vi "Boiler-M.vi"() -> ()   [LabVIEW 2020]
uses:
  Controls/Boiler States Enum-M.ctl
panel:
  in  "stop":bool
  out "Boiler Status Indicators":T1 {"Time Count" format="%.2f"}
  in  "Boiler Simulation Controls":T2 {"Flame Sesnor Value (%)" scale=0.0..100.0}
  in  "Boiler Controls":T3 {"Fuel Control Valve Position (% Open)" scale=0.0..100.0 scale format="%_3g"}
  # "Seconds"
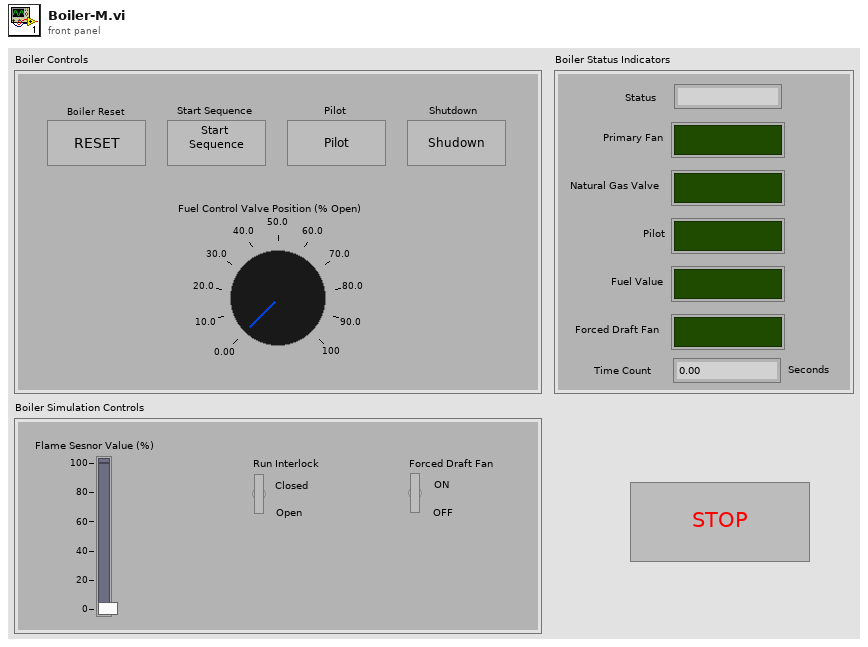
[diagram p1: front panel]
types:
  T1 = cluster{"Primary Fan":bool, "Natural Gas Valve":bool, "Pilot":bool, "Fuel Value":bool, "Forced Draft Fan":bool, "Time Count    ":dbl, "Status":string}
  T2 = cluster{"Flame Sesnor Value (%)":dbl, "Run Interlock":bool, "Forced Draft Fan":bool}
  T3 = cluster{"Shutdown":bool, "Pilot":bool, "Start Sequence":bool, "Fuel Control Valve Position (% Open)":dbl, "Boiler Reset":bool}
  T4 = typedef "Boiler States Enum-M.ctl" = enum16{"Idle", "Initialize", "Reset Lockout", "Pre-Purge", "Pre-Purge Complete", "Ignition", "Pilot", "Shutdown Purge Complete", "Shutdown Purge Start", "Run", "Pilot Proved", "Forced Draft Fan On"}
  T5 = cluster{"Time has Elapsed":bool, "Elapsed Time (s)":dbl}
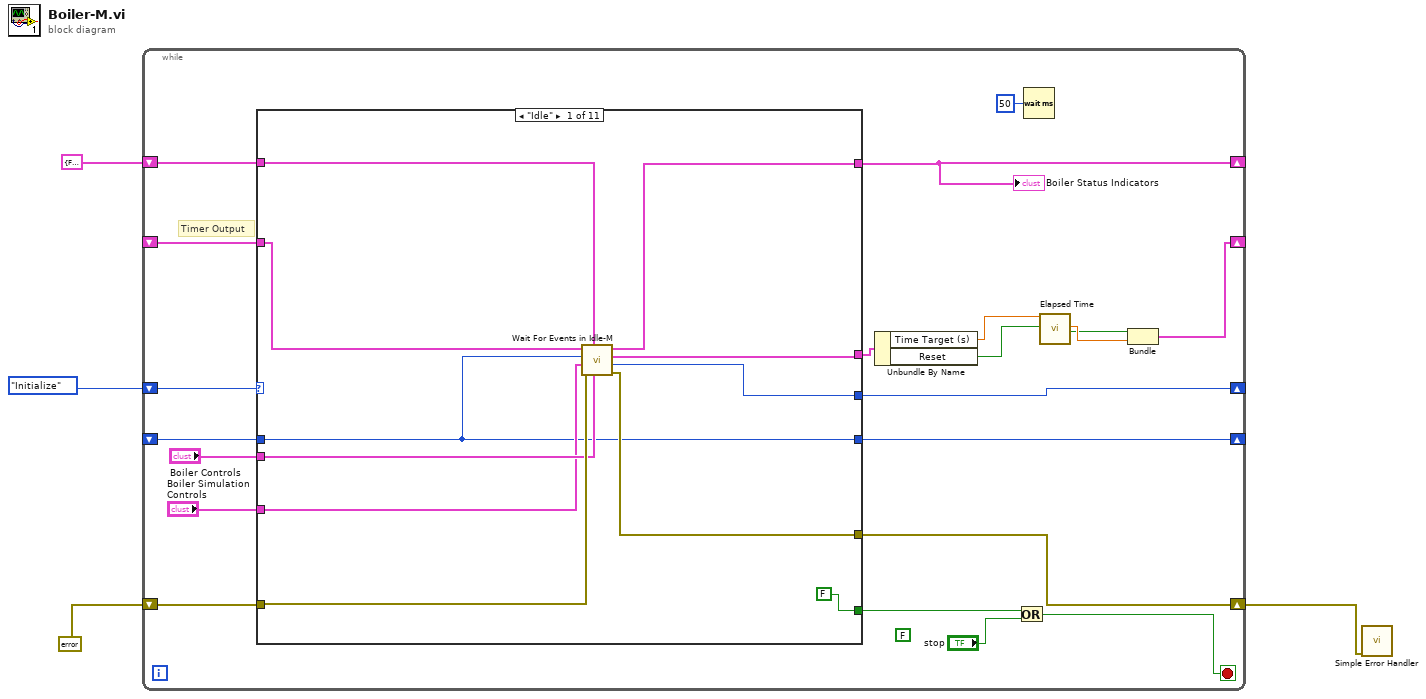
[diagram p0: block diagram]
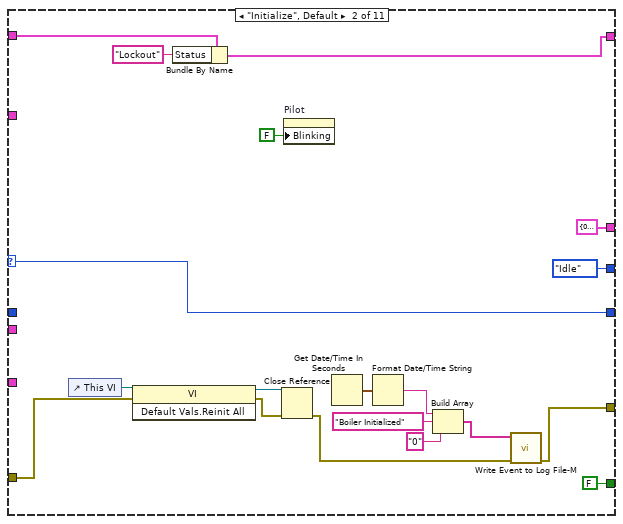
[diagram p2: hidden frame]
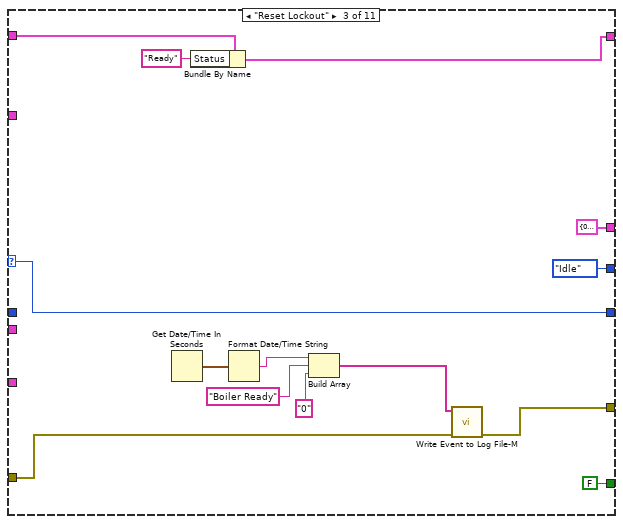
[diagram p3: hidden frame]
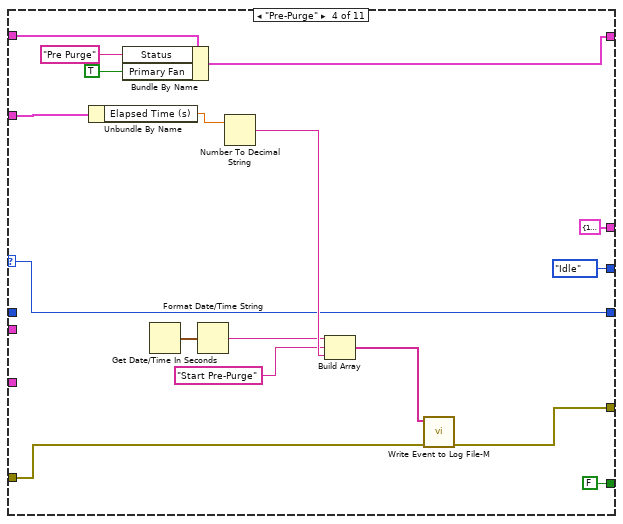
[diagram p4: hidden frame]
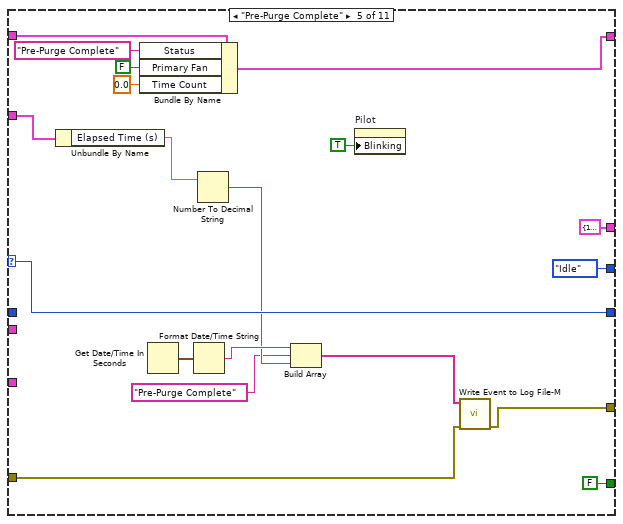
[diagram p5: hidden frame]
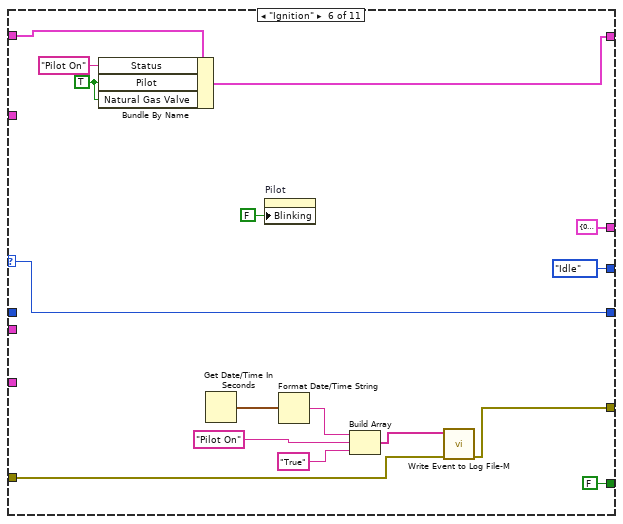
[diagram p6: hidden frame]
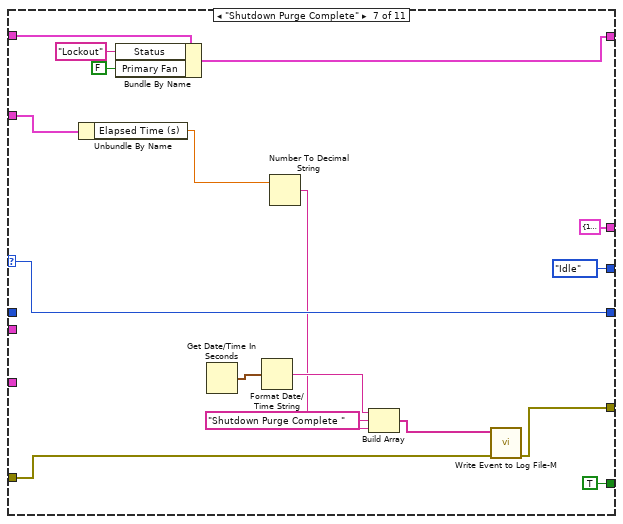
[diagram p7: hidden frame]
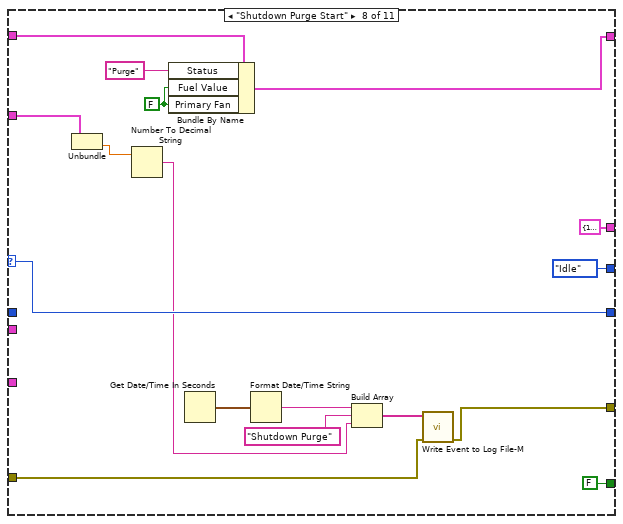
[diagram p8: hidden frame]
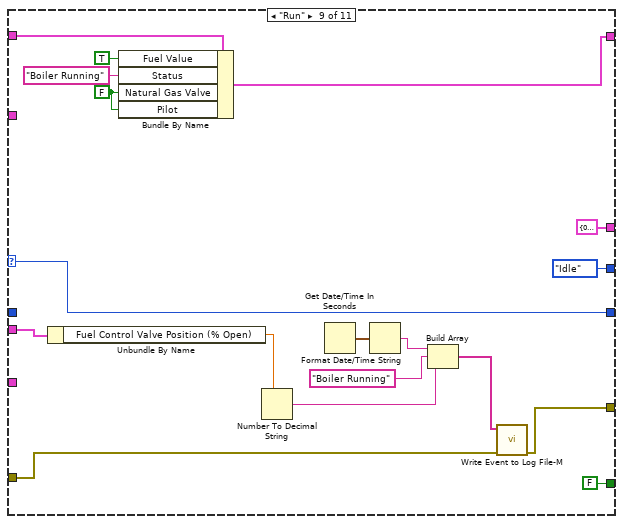
[diagram p9: hidden frame]
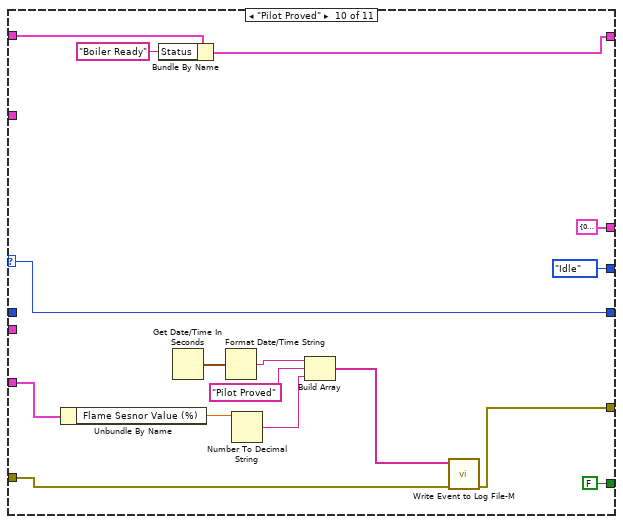
[diagram p10: hidden frame]
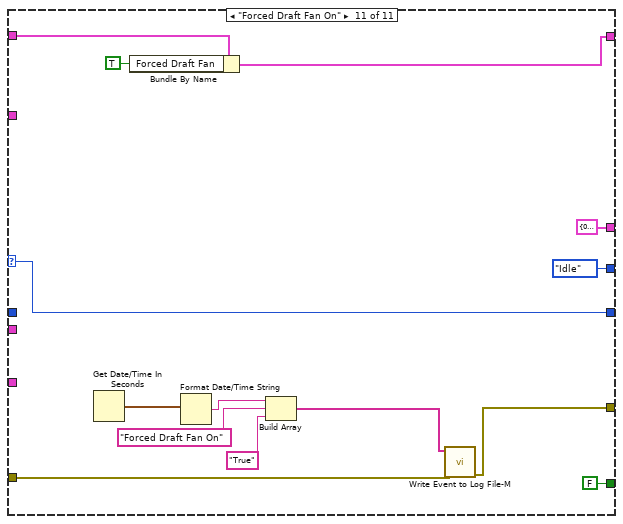
[diagram p11: hidden frame]
diagram:
  n1 = while {
    shift-right: [w24] -> _
    shift-left: T1 {"Primary Fan"=FALSE, "Natural Gas Valve"=FALSE, "Pilot"=FALSE, "Fuel Value"=FALSE, "Forced Draft Fan"=FALSE, "Time Count    "=0.0, "Status"=""} ("Boiler Status Indicators") -> [w25]
    shift-right: [w19] -> _
    shift-left: _ -> [w10]
    shift-right: [w13] -> _
    shift-left: Boiler_States_Enum-M."Initialize" ("Enum") -> [w14]
    shift-right: [w8] -> _
    shift-left: _ -> [w7]
    shift-right: [w9] -> w1
    shift-left: errorcluster {"status"=FALSE, "code"=0, "source"=""} ("error in (no error)") -> [w15]
    stop <- w18 stop-if-true
    (unwired) FALSE
    # "Timer Output"
    n2 = case shown="\"Idle\"" w14 {
      selector: w14 -> [_ w55 w64 w74 w104 w114 w138 w149 w160 w186 w199]
      tunnel: w25 -> [w36 w53 w69 w86 w102 w121 w125 w155 w163 w189 w203]
      tunnel: [w35 w52 w68 w83 w101 w107 w124 w154 w162 w188 w202] -> w24
      tunnel: [w34 cluster{"Time Target (s)":dbl, "Reset":bool} {"Time Target (s)"=0.0, "Reset"=TRUE} ("Cluster out") cluster{"Time Target (s)":dbl, "Reset":bool} {"Time Target (s)"=0.0, "Reset"=TRUE} ("Cluster out") cluster{"Time Target (s)":dbl, "Reset":bool} {"Time Target (s)"=10.0, "Reset"=TRUE} ("Cluster out") cluster{"Time Target (s)":dbl, "Reset":bool} {"Time Target (s)"=10.0, "Reset"=TRUE} ("Cluster out") cluster{"Time Target (s)":dbl, "Reset":bool} {"Time Target (s)"=0.0, "Reset"=TRUE} ("Cluster out") cluster{"Time Target (s)":dbl, "Reset":bool} {"Time Target (s)"=10.0, "Reset"=TRUE} ("Cluster out") cluster{"Time Target (s)":dbl, "Reset":bool} {"Time Target (s)"=10.0, "Reset"=TRUE} ("Cluster out") cluster{"Time Target (s)":dbl, "Reset":bool} {"Time Target (s)"=0.0, "Reset"=TRUE} ("Cluster out") cluster{"Time Target (s)":dbl, "Reset":bool} {"Time Target (s)"=0.0, "Reset"=TRUE} ("Cluster out") cluster{"Time Target (s)":dbl, "Reset":bool} {"Time Target (s)"=0.0, "Reset"=TRUE} ("Cluster out")] -> w22
      tunnel: [FALSE FALSE FALSE FALSE FALSE FALSE TRUE FALSE FALSE FALSE FALSE] -> w16
      tunnel: [w32 w46 w57 w80 w91 w115 w134 w146 w169 w178 w195] -> w9
      tunnel: w15 -> [w31 w49 w63 w79 w90 w116 w133 w140 w167 w179 w196]
      tunnel: [w30 Boiler_States_Enum-M."Idle" ("Next State") Boiler_States_Enum-M."Idle" ("Next State") Boiler_States_Enum-M."Idle" ("Next State") Boiler_States_Enum-M."Idle" ("Next State") Boiler_States_Enum-M."Idle" ("Next State") Boiler_States_Enum-M."Idle" ("Next State") Boiler_States_Enum-M."Idle" ("Next State") Boiler_States_Enum-M."Idle" ("Next State") Boiler_States_Enum-M."Idle" ("Next State") Boiler_States_Enum-M."Idle" ("Next State")] -> w13
      tunnel: "Boiler Controls" -> [w29 _ _ _ _ _ _ _ w172 _ _]
      tunnel: "Boiler Simulation Controls" -> [w28 _ _ _ _ _ _ _ _ w183 _]
      tunnel: w10 -> [w26 _ _ w82 w98 _ w137 w148 _ _ _]
      tunnel: [w27 w55 w64 w74 w104 w114 w138 w149 w160 w186 w199] -> w8
      tunnel: w7 -> [w27 _ _ _ _ _ _ _ _ _ _]
      frame "Idle" {
        n3 = call "Wait For Events in Idle-M.vi"("Boiler Controls"=w29, "Boiler Status Indicators In"=w36, "error in (no error)"=w31, "Boiler Simulation Controls"=w28, "Last State Before Idle"=w27, "Timer Ouput"=w26) -> ("error out"=w32:errorcluster, "Next State"=w30:T4, "Cluster out"=w34:cluster{"Time Target (s)":dbl, "Reset":bool}, "Boiler Status Indicators Out"=w35:T1)  [unwired: 2 in]
      }
      frame "Initialize", Default {
        n4 = control-ref of="This VI"() -> (w37:refnum<vi>)
        n5 = invoke class="VI" method="Default Vals.Reinit All"(reference=w37, error in=w49) -> (reference out=w45:refnum<vi>, error out=w44:errorcluster)  [unwired: 1 in, 1 out]
        n6 = Bundle By Name(cluster=w53, "Status"="Lockout") -> (w52:T1)
        n7 = Close Reference(reference=w45, error in (no error)=w44) -> (error out=w43:errorcluster)
        n8 = property on="Pilot" class="Bool"("Blinking"=FALSE) -> ()  [unwired: 2 in, 2 out]
        n9 = Get Date/Time In Seconds() -> (seconds since 1Jan1904=w38:timestamp)
        n10 = Format Date/Time String(seconds (now)=w38) -> (date/time string=w41:string)  [unwired: 2 in]
        n11 = Build Array(w41, "Boiler Initialized" ("element"), "0" ("element")) -> (w42:string[])
        n12 = call "Write Event to Log File-M.vi"("error in (no error)"=w43, "Array"=w42) -> ("error out"=w46:errorcluster)  [unwired: 9 in]
      }
      frame "Reset Lockout" {
        n13 = Get Date/Time In Seconds() -> (seconds since 1Jan1904=w60:timestamp)
        n14 = Bundle By Name(cluster=w69, "Status"="Ready") -> (w68:T1)
        n15 = Format Date/Time String(seconds (now)=w60) -> (date/time string=w62:string)  [unwired: 2 in]
        n16 = Build Array(w62, "Boiler Ready" ("element"), "0" ("element")) -> (w61:string[])
        n17 = call "Write Event to Log File-M.vi"("error in (no error)"=w63, "Array"=w61) -> ("error out"=w57:errorcluster)  [unwired: 9 in]
      }
      frame "Pre-Purge" {
        n18 = Unbundle By Name(w82) -> ("Elapsed Time (s)"=w70:dbl)
        n19 = Bundle By Name(cluster=w86, "Status"="Pre Purge", "Primary Fan"=TRUE ("Natural Gas Valve")) -> (w83:T1)
        n20 = Get Date/Time In Seconds() -> (seconds since 1Jan1904=w77:timestamp)
        n21 = Format Date/Time String(seconds (now)=w77) -> (date/time string=w76:string)  [unwired: 2 in]
        n22 = Number To Decimal String(number=w70) -> (decimal integer string=w81:string)  [unwired: 1 in]
        n23 = Build Array(w76, "Start Pre-Purge" ("element"), w81) -> (w78:string[])
        n24 = call "Write Event to Log File-M.vi"("error in (no error)"=w79, "Array"=w78) -> ("error out"=w80:errorcluster)  [unwired: 9 in]
      }
      frame "Pre-Purge Complete" {
        n25 = Unbundle By Name(w98) -> ("Elapsed Time (s)"=w97:dbl)
        n26 = Bundle By Name(cluster=w102, "Status"="Pre-Purge Complete", "Primary Fan"=FALSE, "Time Count"=0.0) -> (w101:T1)
        n27 = Get Date/Time In Seconds() -> (seconds since 1Jan1904=w96:timestamp)
        n28 = Format Date/Time String(seconds (now)=w96) -> (date/time string=w95:string)  [unwired: 2 in]
        n29 = Number To Decimal String(number=w97) -> (decimal integer string=w94:string)  [unwired: 1 in]
        n30 = Build Array(w95, "Pre-Purge Complete", w94) -> (w92:string[])
        n31 = property on="Pilot" class="Bool"("Blinking"=TRUE) -> ()  [unwired: 2 in, 2 out]
        n32 = call "Write Event to Log File-M.vi"("error in (no error)"=w90, "Array"=w92) -> ("error out"=w91:errorcluster)  [unwired: 9 in]
      }
      frame "Ignition" {
        w119 = TRUE ("Pilot")
        n33 = Bundle By Name(cluster=w121, "Status"="Pilot On", "Pilot"=w119, "Natural Gas Valve"=w119) -> (w107:T1)
        n34 = Get Date/Time In Seconds() -> (seconds since 1Jan1904=w118:timestamp)
        n35 = property on="Pilot" class="Bool"("Blinking"=FALSE) -> ()  [unwired: 2 in, 2 out]
        n36 = Format Date/Time String(seconds (now)=w118) -> (date/time string=w111:string)  [unwired: 2 in]
        n37 = Build Array(w111, "Pilot On" ("element"), "True" ("element")) -> (w117:string[])
        n38 = call "Write Event to Log File-M.vi"("error in (no error)"=w116, "Array"=w117) -> ("error out"=w115:errorcluster)  [unwired: 9 in]
      }
      frame "Shutdown Purge Complete" {
        n39 = Unbundle By Name(w137) -> ("Elapsed Time (s)"=w136:dbl)
        n40 = Bundle By Name(cluster=w125, "Status"="Lockout", "Primary Fan"=FALSE) -> (w124:T1)
        n41 = Get Date/Time In Seconds() -> (seconds since 1Jan1904=w130:timestamp)
        n42 = Format Date/Time String(seconds (now)=w130) -> (date/time string=w131:string)  [unwired: 2 in]
        n43 = Number To Decimal String(number=w136) -> (decimal integer string=w129:string)  [unwired: 1 in]
        n44 = Build Array(w131, "Shutdown Purge Complete " ("element"), w129) -> (w132:string[])
        n45 = call "Write Event to Log File-M.vi"("error in (no error)"=w133, "Array"=w132) -> ("error out"=w134:errorcluster)  [unwired: 9 in]
      }
      frame "Shutdown Purge Start" {
        w152 = FALSE ("Primary Fan")
        n46 = Unbundle(w148) -> ("Elapsed Time (s)"=w139:dbl)  [unwired: 1 out]
        n47 = Number To Decimal String(number=w139) -> (decimal integer string=w143:string)  [unwired: 1 in]
        n48 = Bundle By Name(cluster=w155, "Status"="Purge", "Fuel Value"=w152, "Primary Fan"=w152) -> (w154:T1)
        n49 = Get Date/Time In Seconds() -> (seconds since 1Jan1904=w142:timestamp)
        n50 = Format Date/Time String(seconds (now)=w142) -> (date/time string=w145:string)  [unwired: 2 in]
        n51 = Build Array(w145, "Shutdown Purge" ("element"), w143) -> (w141:string[])
        n52 = call "Write Event to Log File-M.vi"("error in (no error)"=w140, "Array"=w141) -> ("error out"=w146:errorcluster)  [unwired: 9 in]
      }
      frame "Run" {
        w159 = FALSE ("Natural Gas Valve")
        n53 = Unbundle By Name(w172) -> ("Fuel Control Valve Position (% Open)"=w171:dbl)
        n54 = Bundle By Name(cluster=w163, "Fuel Value"=TRUE, "Status"="Boiler Running", "Natural Gas Valve"=w159, "Pilot"=w159) -> (w162:T1)
        n55 = Number To Decimal String(number=w171) -> (decimal integer string=w165:string)  [unwired: 1 in]
        n56 = Get Date/Time In Seconds() -> (seconds since 1Jan1904=w170:timestamp)
        n57 = Format Date/Time String(seconds (now)=w170) -> (date/time string=w166:string)  [unwired: 2 in]
        n58 = Build Array(w166, "Boiler Running" ("element"), w165) -> (w168:string[])
        n59 = call "Write Event to Log File-M.vi"("error in (no error)"=w167, "Array"=w168) -> ("error out"=w169:errorcluster)  [unwired: 9 in]
      }
      frame "Pilot Proved" {
        n60 = Unbundle By Name(w183) -> ("Flame Sesnor Value (%)"=w182:dbl)
        n61 = Bundle By Name(cluster=w189, "Status"="Boiler Ready") -> (w188:T1)
        n62 = Get Date/Time In Seconds() -> (seconds since 1Jan1904=w181:timestamp)
        n63 = Format Date/Time String(seconds (now)=w181) -> (date/time string=w176:string)  [unwired: 2 in]
        n64 = Number To Decimal String(number=w182) -> (decimal integer string=w174:string)  [unwired: 1 in]
        n65 = Build Array(w176, "Pilot Proved" ("element"), w174) -> (w180:string[])
        n66 = call "Write Event to Log File-M.vi"("error in (no error)"=w179, "Array"=w180) -> ("error out"=w178:errorcluster)  [unwired: 9 in]
      }
      frame "Forced Draft Fan On" {
        n67 = Get Date/Time In Seconds() -> (seconds since 1Jan1904=w192:timestamp)
        n68 = Bundle By Name(cluster=w203, "Forced Draft Fan"=TRUE) -> (w202:T1)
        n69 = Format Date/Time String(seconds (now)=w192) -> (date/time string=w193:string)  [unwired: 2 in]
        n70 = Build Array(w193, "Forced Draft Fan On" ("element"), "True" ("element")) -> (w197:string[])
        n71 = call "Write Event to Log File-M.vi"("error in (no error)"=w196, "Array"=w197) -> ("error out"=w195:errorcluster)  [unwired: 9 in]
      }
    }
    "Boiler Status Indicators" <- w24
    n72 = Unbundle By Name(w22) -> ("Time Target (s)"=w20:dbl, "Reset"=w21:bool)
    n73 = Or(x=w16, y="stop") -> (x .or. y?=w18:bool)
    n74 = Wait (ms)(milliseconds to wait=u32 50) -> ()  [unwired: 1 out]
    n75 = call "Elapsed Time"("Time Target (s)"=w20, "Reset"=w21) -> ("Elapsed Time (s)"=w6:dbl, "Time has Elapsed"=w5:bool)  [unwired: 10 in, 6 out]
    n76 = Bundle("Time has Elapsed"=w5, "Elapsed Time (s)"=w6) -> (w19:T5)  [unwired: 1 in]
  }
  n77 = call <vilib>:"Simple Error Handler.vi"("error in (no error)"=w1) -> ()  [unwired: 4 in, 5 out]
